vi "Checking_connection2.vi"(8 "error in":errorcluster, 11 "paramUnicornIn":T2={"conParam"={"ReadIntParam"=TRUE, "ReadDescrParam"=FALSE, "ReadFloatParam"=TRUE, "debug"=FALSE, "ReadJSON"=TRUE, "IP_address"="192.168.1.216", "N_attempts"=3, "type_con"=enum."TCP", "MB_address"=1, "VISA"="COM1", "connection ID"=refnum, "nameDevices"="", "timeout"=3000, "port"=2000, "type_version"="0F0C0001", "baud_rate"=115200, "VersionControl"=TRUE, "TCP_conn"=TRUE, "WindowSize"=700}, "Param"={"NumParam"={"NTelem"=201, "NInt"=16, "NFloat"=10, "NTable"=2}, "ParamInt"=[{"ID"="Режим работы", "Num"=0, "Name"="", "Type"="", "Enum"="", "Desc"="", "Unit"="", "Access"="", "FormatStr"="", "Min"=0, "Max"=0}, {"ID"="", "Num"=0, "Name"="", "Type"="", "Enum"="", "Desc"="", "Unit"="", "Access"="", "FormatStr"="", "Min"=0, "Max"=0}, {"ID"="", "Num"=0, "Name"="", "Type"="", "Enum"="", "Desc"="", "Unit"="", "Access"="", "FormatStr"="", "Min"=0, "Max"=0}, {"ID"="", "Num"=0, "Name"="", "Type"="", "Enum"="", "Desc"="", "Unit"="", "Access"="", "FormatStr"="", "Min"=0, "Max"=0}, {"ID"="", "Num"=0, "Name"="", "Type"="", "Enum"="", "Desc"="", "Unit"="", "Access"="", "FormatStr"="", "Min"=0, "Max"=0}, {"ID"="", "Num"=0, "Name"="", "Type"="", "Enum"="", "Desc"="", "Unit"="", "Access"="", "FormatStr"="", "Min"=0, "Max"=0}, {"ID"="ModeWork", "Num"=0, "Name"="", "Type"="", "Enum"="", "Desc"="", "Unit"="", "Access"="", "FormatStr"="", "Min"=0, "Max"=0}], "Telemetry"=[], "Table"=[], "ParamFloat"=[]}}) -> (0 "error out":errorcluster, 1 "conParam.TCP_conn":bool, 2 "ArrayData":T9, 3 "paramUnicorn":T2={"conParam"={"ReadIntParam"=TRUE, "ReadDescrParam"=FALSE, "ReadFloatParam"=TRUE, "debug"=FALSE, "ReadJSON"=TRUE, "IP_address"="192.168.1.216", "N_attempts"=3, "type_con"=enum."TCP", "MB_address"=1, "VISA"="COM1", "connection ID"=refnum, "nameDevices"="", "timeout"=3000, "port"=2000, "type_version"="0F0C0001", "baud_rate"=115200, "VersionControl"=TRUE, "TCP_conn"=TRUE, "WindowSize"=700}, "Param"={"NumParam"={"NTelem"=201, "NInt"=16, "NFloat"=10, "NTable"=2}, "ParamInt"=[{"ID"="Режим работы", "Num"=0, "Name"="", "Type"="", "Enum"="", "Desc"="", "Unit"="", "Access"="", "FormatStr"="", "Min"=0, "Max"=0}, {"ID"="", "Num"=0, "Name"="", "Type"="", "Enum"="", "Desc"="", "Unit"="", "Access"="", "FormatStr"="", "Min"=0, "Max"=0}, {"ID"="", "Num"=0, "Name"="", "Type"="", "Enum"="", "Desc"="", "Unit"="", "Access"="", "FormatStr"="", "Min"=0, "Max"=0}, {"ID"="", "Num"=0, "Name"="", "Type"="", "Enum"="", "Desc"="", "Unit"="", "Access"="", "FormatStr"="", "Min"=0, "Max"=0}, {"ID"="", "Num"=0, "Name"="", "Type"="", "Enum"="", "Desc"="", "Unit"="", "Access"="", "FormatStr"="", "Min"=0, "Max"=0}, {"ID"="", "Num"=0, "Name"="", "Type"="", "Enum"="", "Desc"="", "Unit"="", "Access"="", "FormatStr"="", "Min"=0, "Max"=0}, {"ID"="ModeWork", "Num"=0, "Name"="", "Type"="", "Enum"="", "Desc"="", "Unit"="", "Access"="", "FormatStr"="", "Min"=0, "Max"=0}], "Telemetry"=[], "Table"=[], "ParamFloat"=[]}})   [LabVIEW 2017, in "LV_Unicorn.lvlib"]
uses:
  LV_Unicorn.lvlib
  Control/unicorn_Param.ctl
  Control/unicorn_conn.ctl
  Control/unicorn_JSON.ctl
  Control/unicorn_ParamInt.ctl
  Control/unicorn_Telemetry.ctl
  Control/unicorn_Table.ctl
  Control/unicorn_ParamFloat.ctl
  Control/unicorn_array.ctl
  <vilib>/Utility/error.llb/DialogType.ctl
panel:
  out "Тип/версия устройства":string
  in  "Tab Control":T1(tab)
  out "JSONStr":string
  # "Подключение к устройству"
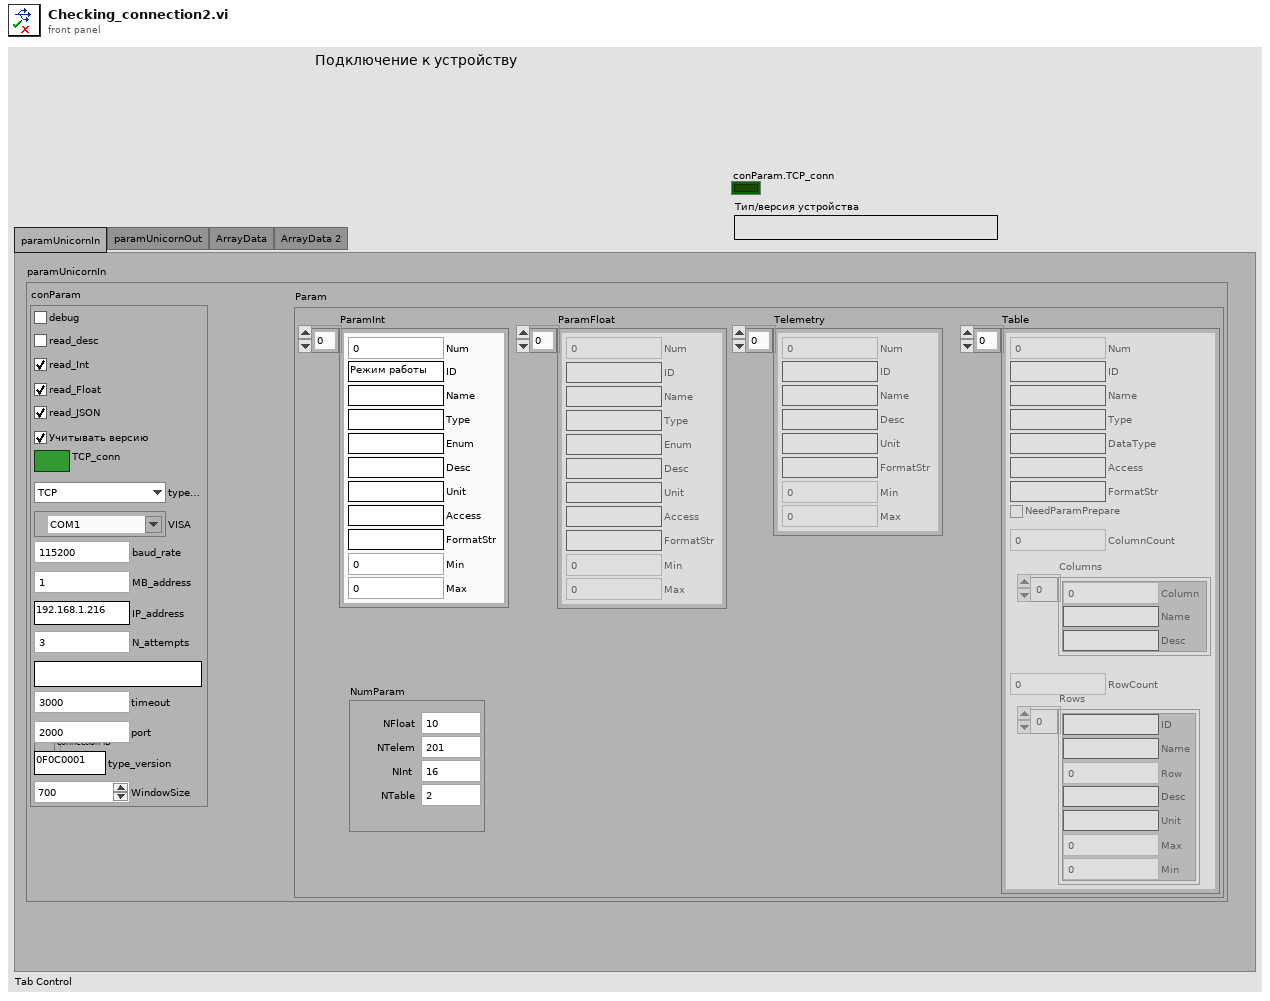
[diagram p1: front panel]
types:
  T1 = enum32{"paramUnicornIn", "paramUnicornOut", "ArrayData", "ArrayData 2"}
  T2 = typedef "LV_Unicorn.lvlib/unicorn_Param.ctl" = cluster{"conParam":T3, "Param":T4}
  T3 = typedef "LV_Unicorn.lvlib/unicorn_conn.ctl" = cluster{"ReadIntParam":bool, "ReadDescrParam":bool, "ReadFloatParam":bool, "debug":bool, "ReadJSON":bool, "IP_address":string, "N_attempts":i32, "type_con":enum16{"Serial", "TCP"}, "MB_address":i32, "VISA":refnum<visa-resource-name>, "connection ID":refnum<k5>, "nameDevices":string, "timeout":i32, "port":u16, "type_version":string, "baud_rate":u32, "VersionControl":bool, "TCP_conn":bool, "WindowSize":i32}
  T4 = typedef "LV_Unicorn.lvlib/unicorn_JSON.ctl" = cluster{"NumParam":cluster{"NTelem":i32, "NInt":i32, "NFloat":i32, "NTable":i32}, "ParamInt":T5, "Telemetry":T6, "Table":T7, "ParamFloat":T8}
  T5 = typedef "LV_Unicorn.lvlib/unicorn_ParamInt.ctl" = cluster{"ID":string, "Num":i32, "Name":string, "Type":string, "Enum":string, "Desc":string, "Unit":string, "Access":string, "FormatStr":string, "Min":i32, "Max":i32}[]
  T6 = typedef "LV_Unicorn.lvlib/unicorn_Telemetry.ctl" = cluster{"ID":string, "Num":i32, "Name":string, "Desc":string, "Unit":string, "FormatStr":string, "Min":i32, "Max":i32}[]
  T7 = typedef "LV_Unicorn.lvlib/unicorn_Table.ctl" = cluster{"Num":i32, "Access":string, "ColumnCount":i32, "NeedParamPrepare":bool, "Columns":cluster{"Column":i32, "Desc":string, "Name":string}[], "DataType":string, "FormatStr":string, "ID":string, "Name":string, "RowCount":i32, "Rows":cluster{"Desc":string, "ID":string, "Max":i32, "Min":i32, "Name":string, "Row":i32, "Unit":string}[], "Type":string}[]
  T8 = typedef "LV_Unicorn.lvlib/unicorn_ParamFloat.ctl" = cluster{"ID":string, "Num":i32, "Name":string, "Type":string, "Enum":string, "Desc":string, "Unit":string, "Access":string, "FormatStr":string, "Min":sgl, "Max":sgl}[]
  T9 = typedef "LV_Unicorn.lvlib/unicorn_array.ctl" = cluster{"ArrayInt":i32[], "ArrayFloat":sgl[], "Telemetry":sgl[]}
  T10 = typedef "DialogType.ctl" = u16
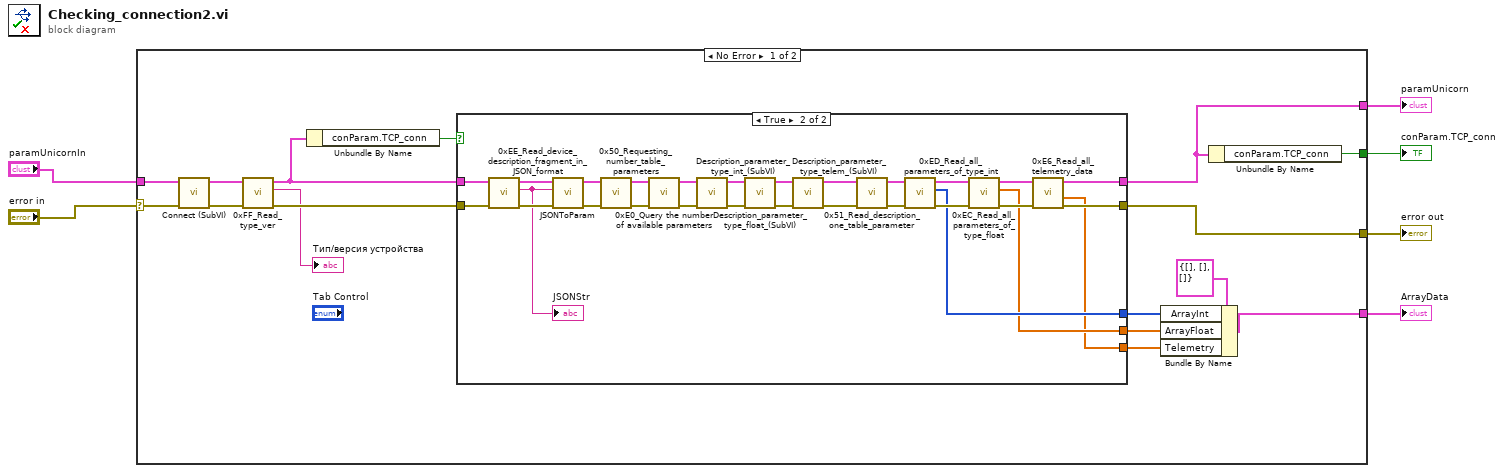
[diagram p0: block diagram]
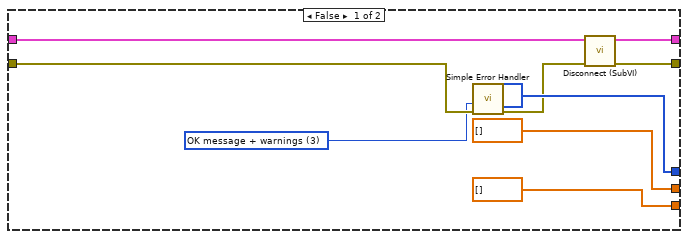
[diagram p2: hidden frame]
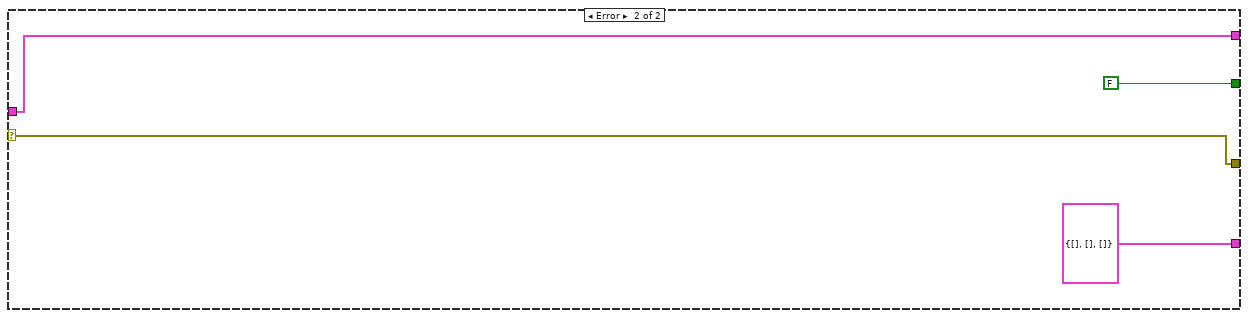
[diagram p3: hidden frame]
diagram:
  n1 = case shown="No Error" "error in" {
    selector: "error in" -> [w8 w61]
    tunnel: [w22 w61] -> w6
    tunnel: "paramUnicornIn" -> [w21 w62]
    tunnel: [w16 T9 {"ArrayInt"=[], "ArrayFloat"=[], "Telemetry"=[]} ("ArrayUnicorn")] -> w4
    tunnel: [w10 w62] -> w3
    tunnel: [w9 FALSE ("TCP_conn")] -> w2
    frame No Error {
      n2 = call "Connect (SubVI).vi"("error in (no error)"=w8, "paramUnicornIn"=w21) -> ("error out"=w14:errorcluster, "paramUnicornIn out"=w15:T2)  [unwired: 8 in]
      n3 = call "0xFF_Read_type_ver.vi"("error in (no error)"=w14, "paramUnicornIn in"=w15) -> ("error out"=w12:errorcluster, "Тип/версия устройства"=→"Тип/версия устройства":string, "paramUnicornIn out 2"=w13:T2)  [unwired: 7 in]
      n4 = Unbundle By Name(w13) -> ("conParam.TCP_conn"=w11:bool)
      n5 = case shown="True" w11 {
        tunnel: [w26 w51] -> w22
        tunnel: [w27 w52] -> w10
        tunnel: [i32[] [] ("ArrayInt") w50] -> w19
        tunnel: [sgl[] [] ("ArrayFloat") w49] -> w18
        tunnel: [sgl[] [] ("Telemetry") w48] -> w17
        tunnel: w13 -> [w28 w47]
        tunnel: w12 -> [w25 w46]
        frame False {
          w23 = T10 3 items=["no dialog", "OK message", "continue or stop message", "OK message + warnings", "continue/stop + warnings"] ("type of dialog (OK msg:1)")
          n6 = call <vilib>:"Simple Error Handler.vi"("type of dialog (OK msg:1)"=w23, "error in (no error)"=w25) -> ("error out"=w24:errorcluster)  [unwired: 3 in, 4 out]
          n7 = call "Disconnect (SubVI).vi"("error in (no error)"=w24, "paramUnicornIn"=w28) -> ("error out"=w26:errorcluster, "paramUnicornIn 2"=w27:T2)  [unwired: 8 in]
        }
        frame True {
          n8 = call "0xEE_Read_device_description_fragment_in_JSON_format.vi"("error in"=w46, "paramUnicorn 2"=w47) -> ("error out"=w59:errorcluster, "JSONStr"=w57:string, "paramUnicorn"=w58:T2)  [unwired: 7 in]
          "JSONStr" <- w57
          n9 = call "JSONToParam.vi"("error in"=w59, "JSON"=w57, "paramUnicornIn"=w58) -> ("error out"=w44:errorcluster, "paramUnicornOut"=w45:T2)  [unwired: 7 in]
          n10 = call "0x50_Requesting_number_table_parameters.vi"("error in"=w44, "paramUnicorn"=w45) -> ("error out"=w42:errorcluster, "paramUnicorn 2"=w43:T2)  [unwired: 8 in]
          n11 = call "0xE0_Query the number of available parameters.vi"("error in"=w42, "paramUnicorn"=w43) -> ("error out"=w41:errorcluster, "paramUnicorn out"=w40:T2)  [unwired: 8 in]
          n12 = call "Description_parameter_type_int_(SubVI).vi"("error in (no error)"=w41, "paramUnicorn in"=w40) -> ("error out"=w39:errorcluster, "paramUnicornIn out 2"=w38:T2)  [unwired: 8 in]
          n13 = call "Description_parameter_type_float_(SubVI).vi"("error in (no error)"=w39, "paramUnicorn in"=w38) -> ("error out"=w36:errorcluster, "paramUnicornIn out 2"=w37:T2)  [unwired: 8 in]
          n14 = call "Description_parameter_type_telem_(SubVI).vi"("error in (no error)"=w36, "paramUnicorn in"=w37) -> ("error out"=w35:errorcluster, "paramUnicornIn out 2"=w34:T2)  [unwired: 8 in]
          n15 = call "0x51_Read_description_one_table_parameter.vi"("error in"=w35, "paramUnicornIn in"=w34) -> ("error out"=w32:errorcluster, "paramUnicornIn out 2"=w33:T2)  [unwired: 8 in]
          n16 = call "0xED_Read_all_parameters_of_type_int.vi"("error in"=w32, "paramUnicorn"=w33) -> ("error out"=w55:errorcluster, "ArrayInt"=w50:i32[], "paramUnicorn 2"=w56:T2)  [unwired: 6 in, 1 out]
          n17 = call "0xEC_Read_all_parameters_of_type_float.vi"("error in"=w55, "paramUnicorn"=w56) -> ("error out"=w53:errorcluster, "ArrayFloat"=w49:sgl[], "paramUnicorn 2"=w54:T2)  [unwired: 6 in, 1 out]
          n18 = call "0xE6_Read_all_telemetry_data.vi"("error in"=w53, "paramUnicorn"=w54) -> ("error out"=w51:errorcluster, "Telemetry"=w48:sgl[], "paramUnicorn 2"=w52:T2)  [unwired: 5 in, 1 out]
        }
      }
      n19 = Bundle By Name(cluster=T9 {"ArrayInt"=[], "ArrayFloat"=[], "Telemetry"=[]} ("ArrayUnicorn"), "ArrayInt"=w19, "ArrayFloat"=w18, "Telemetry"=w17) -> (w16:T9)
      n20 = Unbundle By Name(w10) -> ("conParam.TCP_conn"=w9:bool)
    }
    frame Error {
    }
  }
  "error out" <- w6
  "paramUnicorn" <- w3
  "ArrayData" <- w4
  "conParam.TCP_conn" <- w2
